vi "GetObjHelp.vi"(8 "error in (no error)":errorcluster, 11 "GObject in":refnum<class "GObject.lvclass">) -> (0 "error out":errorcluster, 1 "help tag":string, 2 "help path":path, 3 "GObject out":refnum<class "GObject.lvclass">, 4 "has example":bool)   [LabVIEW 2015, in "GObject.lvclass"]
doc: "Returns the help information for the object.\n\nQControl Class wrapper around the <b>GObject : Get Help Info Method</b>.\n<b> </b> <b> </b>\n©2016 Q Software Innovations, LLC (QSI)\nwritten by Quentin Alldredge\nproduced in LabVIEW 2015\n\nsupport@qsoftwareinnovations.com\nwww.qsoftwareinnovations.com\n\nAll rights reserved.\n\nRedistribution and use in source and binary forms, with or without modification, are permitted provided that the following conditions are met:\n\n * Redistributions of source code must retain the above copyright notice, this list of conditions and the following disclaimer.\n * Redistributions in binary form must reproduce the above copyright notice, this list of conditions and the following disclaimer in the documentation and/or other materials provided with the distribution.\n * Neither the name of Q Software Innovations, LLC. nor the names of its contributors may be used to endorse or promote products derived from this software without specific prior written permission.\n\nTHIS SOFTWARE IS PROVIDED BY THE COPYRIGHT HOLDERS AND CONTRIBUTORS \"AS IS\" AND ANY EXPRESS OR IMPLIED WARRANTIES, INCLUDING, BUT NOT LIMITED TO, THE IMPLIED WARRANTIES OF MERCHANTABILITY AND FITNESS FOR A PARTICULAR PURPOSE ARE DISCLAIMED. IN NO EVENT SHALL THE COPYRIGHT OWNER OR CONTRIBUTORS BE LIABLE FOR ANY DIRECT, INDIRECT, INCIDENTAL, SPECIAL, EXEMPLARY, OR CONSEQUENTIAL DAMAGES (INCLUDING, BUT NOT LIMITED TO, PROCUREMENT OF SUBSTITUTE GOODS OR SERVICES; LOSS OF USE, DATA, OR PROFITS; OR BUSINESS INTERRUPTION) HOWEVER CAUSED AND ON ANY THEORY OF LIABILITY, WHETHER IN CONTRACT, STRICT LIABILITY, OR TORT (INCLUDING NEGLIGENCE OR OTHERWISE) ARISING IN ANY WAY OUT OF THE USE OF THIS SOFTWARE, EVEN IF ADVISED OF THE POSSIBILITY OF SUCH DAMAGE."
uses:
  GObject.lvclass
  GObject.lvclass/GObject.ctl
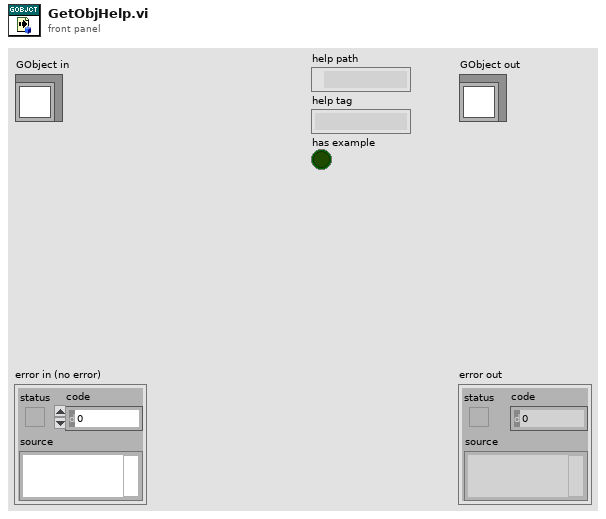
[diagram p1: front panel]
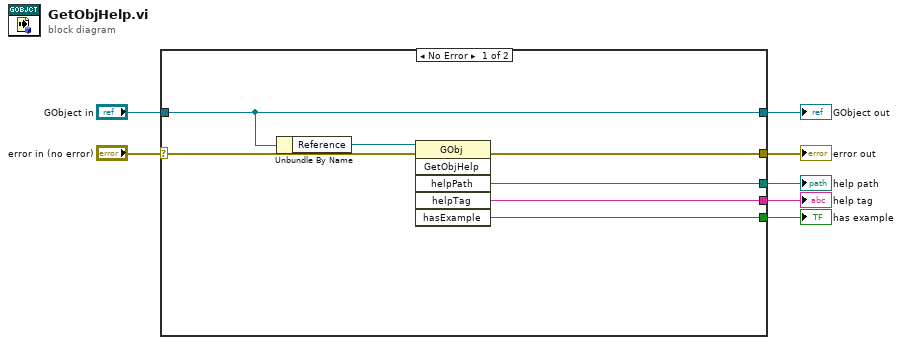
[diagram p0: block diagram]
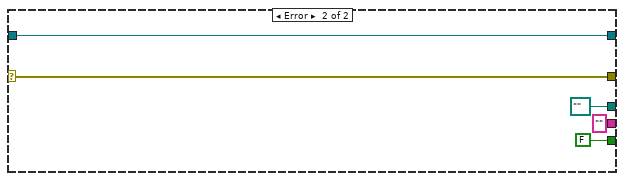
[diagram p2: hidden frame]
diagram:
  n1 = case shown="No Error" "error in (no error)" {
    selector: "error in (no error)" -> [w14 w19]
    tunnel: [w13 w19] -> w6
    tunnel: [w12 w18] -> w4
    tunnel: "GObject in" -> [w12 w18]
    tunnel: [w10 path "" ("helpPath")] -> w3
    tunnel: [w9 "" ("helpTag")] -> w2
    tunnel: [w8 FALSE ("hasExample")] -> w1
    frame No Error {
      n2 = Unbundle By Name(w12) -> ("Reference"=w11:refnum<vi>)
      n3 = invoke class="GObj" method="GetObjHelp"(reference=w11, error in=w14) -> (error out=w13:errorcluster, "helpPath"=w10:path, "helpTag"=w9:string, "hasExample"=w8:bool)  [unwired: 4 in, 2 out]
    }
    frame Error {
    }
  }
  "error out" <- w6
  "GObject out" <- w4
  "help path" <- w3
  "help tag" <- w2
  "has example" <- w1
